vi "sedSpectrometer_salEvent_Timeout.vi"(8 "error in (no error)":errorcluster) -> (0 "error out":errorcluster, 3 "function return":i32)   [LabVIEW 2016, in "SALLV_sedSpectrometer.lvlib"]
doc: "int sedSpectrometer_shm_salEvent_TimeoutLV();"
uses:
  SALLV_sedSpectrometer.lvlib
  SALLV_sedSpectrometer.so
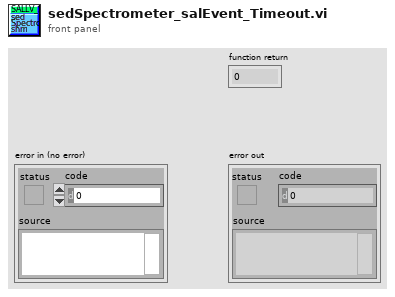
[diagram p1: front panel]
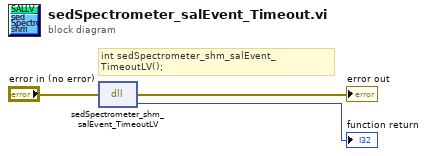
[diagram p0: block diagram]
diagram:
  # "int sedSpectrometer_shm_salEvent_TimeoutLV();"
  n1 = dll-call lib="home/harini/TCS/SALLV_sedSpectrometer/SALLV_sedSpectrometer.*" fn="sedSpectrometer_shm_salEvent_TimeoutLV"(error in="error in (no error)") -> (error out=→"error out":errorcluster, →"function return":i32)  [unwired: 2 in, 1 out]
